vi "Run_Close VI.vi"(6 "DO?":enum16{"Run", "Stop"}(ring), 8 "error in (no error)":errorcluster, 10 "Ref In":refnum<k7>, 11 "VI Parh":path) -> (0 "error out":errorcluster)   [LabVIEW 2018]
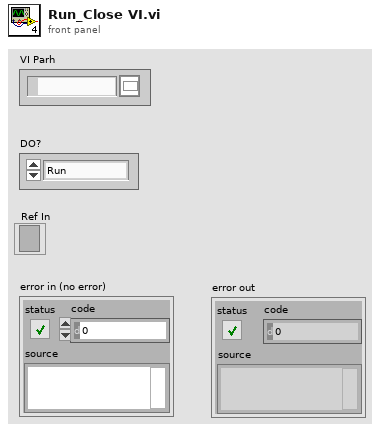
[diagram p1: front panel]
types:
  T1 = enum32{"Bad", "Idle", "Run top level", "Running"}
  T2 = enum32{"Invalid", "Standard", "Closed", "Hidden", "Minimized", "Maximized"}
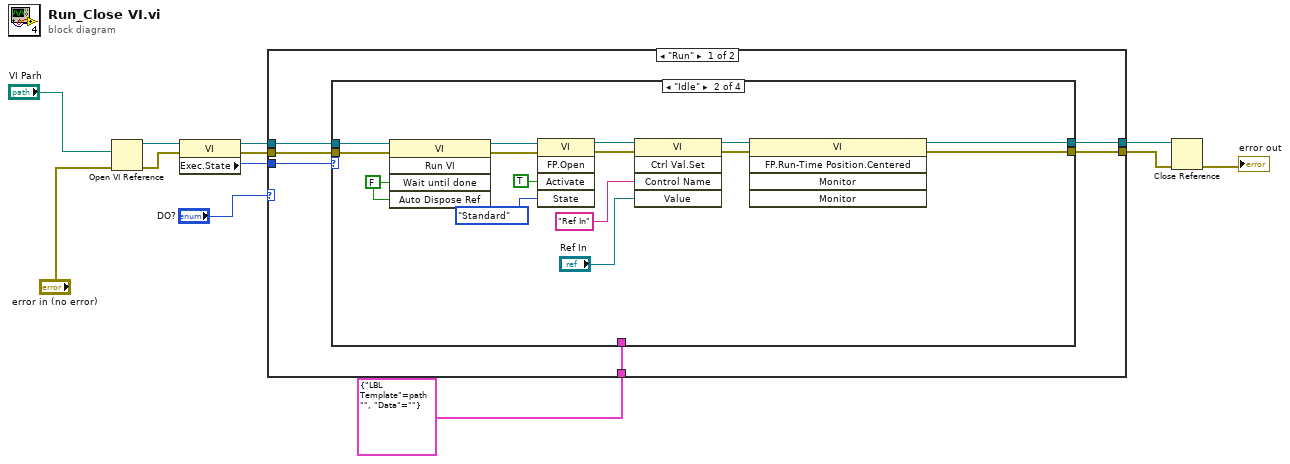
[diagram p0: block diagram]
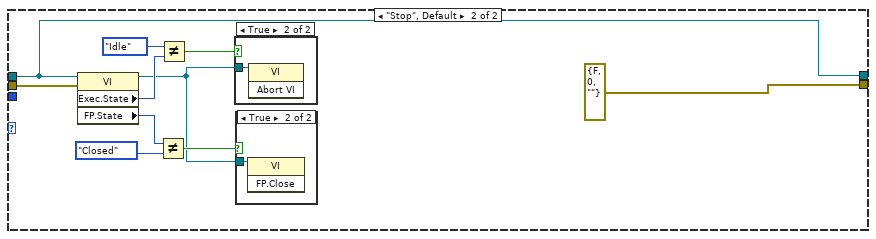
[diagram p5: hidden frame]
diagram:
  n1 = Open VI Reference(vi path="VI Parh", error in (no error)="error in (no error)") -> (vi reference=w5:refnum<vi>, error out=w9:errorcluster)  [unwired: 4 in]
  n2 = property class="VI"(reference=w5, error in=w9) -> (reference out=w8:refnum<vi>, error out=w7:errorcluster, "Exec.State"=w6:T1)
  n3 = case shown="\"Run\"" "DO?" {
    tunnel: [w18 w41] -> w11
    tunnel: [w17 errorcluster {"status"=FALSE, "code"=0, "source"=""} ("error in (no error)")] -> w10
    tunnel: w8 -> [w16 w41]
    tunnel: w7 -> [w15 w49]
    tunnel: w6 -> [w14 _]
    tunnel: cluster{"LBL Template":path, "Data":string} {"LBL Template"=path "", "Data"=""} -> [w13 _]
    frame "Run" {
      n4 = case shown="\"Idle\"" w14 {
        tunnel: w16 -> [w20 w35 w37 w39]
        tunnel: w15 -> [w19 w34 w36 w38]
        tunnel: [w20 w28 w37 w39] -> w18
        tunnel: [w19 w27 w36 w38] -> w17
        tunnel: w13 -> [_ _ _ _]
        frame "Bad", Default {
        }
        frame "Idle" {
          w33 = FALSE ("Wait Until Done")
          n5 = invoke class="VI" method="Run VI"(reference=w35, error in=w34, "Wait until done"=w33, "Auto Dispose Ref"=w33) -> (reference out=w32:refnum<vi>, error out=w31:errorcluster)  [unwired: 1 in, 3 out]
          n6 = invoke class="VI" method="FP.Open"(reference=w32, error in=w31, "Activate"=TRUE ("Activate?"), "State"=T2."Standard") -> (reference out=w22:refnum<vi>, error out=w26:errorcluster)  [unwired: 1 in, 3 out]
          n7 = invoke class="VI" method="Ctrl Val.Set"(reference=w22, error in=w26, "Control Name"="Ref In", "Value"="Ref In") -> (reference out=w25:refnum<vi>, error out=w24:errorcluster)  [unwired: 1 in, 3 out]
          n8 = invoke class="VI" method="FP.Run-Time Position.Centered"(reference=w25, error in=w24) -> (reference out=w28:refnum<vi>, error out=w27:errorcluster)  [unwired: 3 in, 3 out]
        }
        frame "Run top level" {
        }
        frame "Running" {
        }
      }
    }
    frame "Stop", Default {
      n9 = property class="VI"(reference=w41, error in=w49) -> (reference out=w42:refnum<vi>, "Exec.State"=w45:T1, "FP.State"=w48:T2)  [unwired: 1 out]
      n10 = Not Equal?(x=w48, y=T2."Closed") -> (x != y?=w46:bool)
      n11 = Not Equal?(x=T1."Idle", y=w45) -> (x != y?=w43:bool)
      n12 = case shown="True" w43 {
        tunnel: w42 -> [_ w50]
        frame False {
        }
        frame True {
          n13 = invoke class="VI" method="Abort VI"(reference=w50) -> ()  [unwired: 2 in, 3 out]
        }
      }
      n14 = case shown="True" w46 {
        tunnel: w42 -> [_ w51]
        frame False {
        }
        frame True {
          n15 = invoke class="VI" method="FP.Close"(reference=w51) -> ()  [unwired: 2 in, 3 out]
        }
      }
    }
  }
  n16 = Close Reference(reference=w11, error in (no error)=w10) -> (error out=→"error out":errorcluster)
